vi "Vector_place.vi"(11 "vector":cluster{"length":dbl, "angle":dbl}) -> (3 "x,y":cluster{dbl, dbl})   [LabVIEW 2024]
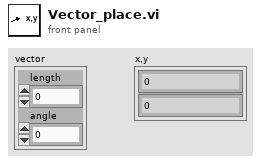
[diagram p1: front panel]
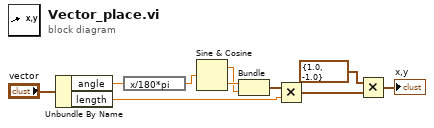
[diagram p0: block diagram]
diagram:
  n1 = Unbundle By Name("vector") -> ("angle"=w10:dbl, "length"=w8:dbl)
  n2 = expression code="x/180*pi"(w10) -> (w4:dbl)
  n3 = Sine & Cosine(0:w4) -> (1:w5:dbl, 2:w6:dbl)
  n4 = Bundle(w6, w5) -> (w7:cluster{dbl, dbl})  [unwired: 1 in]
  n5 = Multiply(x=w7, y=w8) -> (x*y=w9:cluster{dbl, dbl})
  n6 = Multiply(x=cluster{"x":dbl, "y":dbl} {"x"=1.0, "y"=-1.0} ("vector"), y=w9) -> (x*y=→"x,y":cluster{dbl, dbl})
